vi "LVObject to JSON - Descendant Class - Returns JSON Object With All Fields.vi"() -> ()   [LabVIEW 2017, in "Generic Object Serializer Tests.lvlib"]
uses:
  Generic Object Serializer Tests.lvlib
  Generic Object Serializer/Generic Object Serializer.lvclass
  Temperature Forecast/Temperature Forecast.lvclass
  <vilib>/addons/_JKI Toolkits/Caraya/classes/Assert/Assert Equal Value_Variant.vi
  <vilib>/addons/_JKI Toolkits/Caraya/classes/Test/Test.lvclass
  <vilib>/addons/_JKI Toolkits/Caraya/classes/Assert/Assert.lvclass
panel:
  out "error out":errorcluster
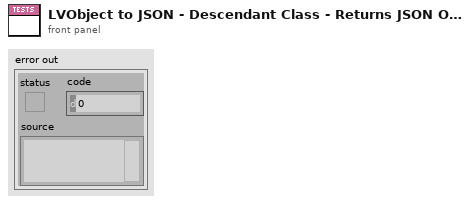
[diagram p1: front panel]
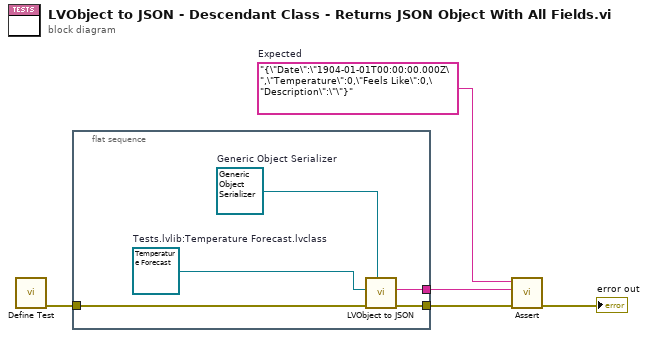
[diagram p0: block diagram]
diagram:
  w1 = "{\"Date\":\"1904-01-01T00:00:00.000Z\",\"Temperature\":0,\"Feels Like\":0,\"Description\":\"\"}"  # Expected
  n1 = call <vilib>:"Define Test.vi"() -> ("error out"=w4:errorcluster)  [unwired: 11 in]
  n2 = flat-sequence {
    tunnel: w4 -> [w9]
    tunnel: [w8] -> w3
    tunnel: [w6] -> w2
    frame #0 {
      w7 = refnum<class "Temperature Forecast.lvclass"> refnum  # Tests.lvlib:Temperature Forecast.lvclass
      w10 = refnum<class "Generic Object Serializer.lvclass"> refnum  # Generic Object Serializer
      n3 = call-dynamic "LVObject to JSON.vi"("LVClass Serializer"=w10, "error in (no error)"=w9, "Object"=w7) -> ("error out"=w8:errorcluster, "<JSON>Object"=w6:string)  [unwired: 7 in]
    }
  }
  n4 = call-poly <vilib>:"Assert.vi"("error in (no error)"=w3, "Y"=w2, "X"=w1) -> ("error out"=→"error out":errorcluster)  [unwired: 8 in]
